vi "HB_Society.Main.vi"() -> ()   [LabVIEW 2009, in "HB_BaseClass_Examples.lvlib"]
doc: "This is a VI to test the simple composition without usage of the Visitor Pattern.\n\nIt demonstrates how to build a continent with contries and towns."
uses:
  HB_BaseClass_Examples.lvlib
  HB_Factory/HB_Factory.lvclass
  HB_Society.lvclass
  lib.lib/HGF_LVC/HGF_BaseClasses/HGF_Factory/HGF_Factory.lvclass
  lib.lib/HGF_LVC/HGF_BaseClasses/HGF_Composite/HGF_Composite.lvclass
panel:
  out "objects":T1(array[cluster])
  out "nofPersons 3":dbl
  out "nofPersons 2":dbl
  out "nofPersons 1":dbl
  in  "Continent":string="Europe"
  in  "Countries":T2(array[cluster])=[{"Name"="Germany", "Towns"=[{"Name"="Essen", "nofPersons"=300}, {"Name"="Bochum", "nofPersons"=200}, {"Name"="Darmstadt", "nofPersons"=200}]}, {"Name"="Montenegro", "Towns"=[{"Name"="Podgorica", "nofPersons"=300}, {"Name"="Bar", "nofPersons"=200}, {"Name"="Ulcinj", "nofPersons"=100}]}]
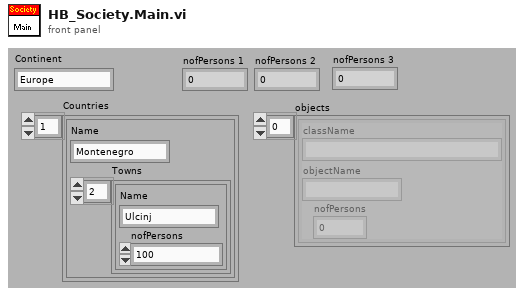
[diagram p1: front panel]
types:
  T1 = cluster{"className":string, "objectName":string, "nofPersons":dbl}[]
  T2 = cluster{"Name":string, "Towns":cluster{"Name":string, "nofPersons":i32}[]}[]
  T3 = cluster{"className":string, "objectName":string, "nofPersons":dbl}
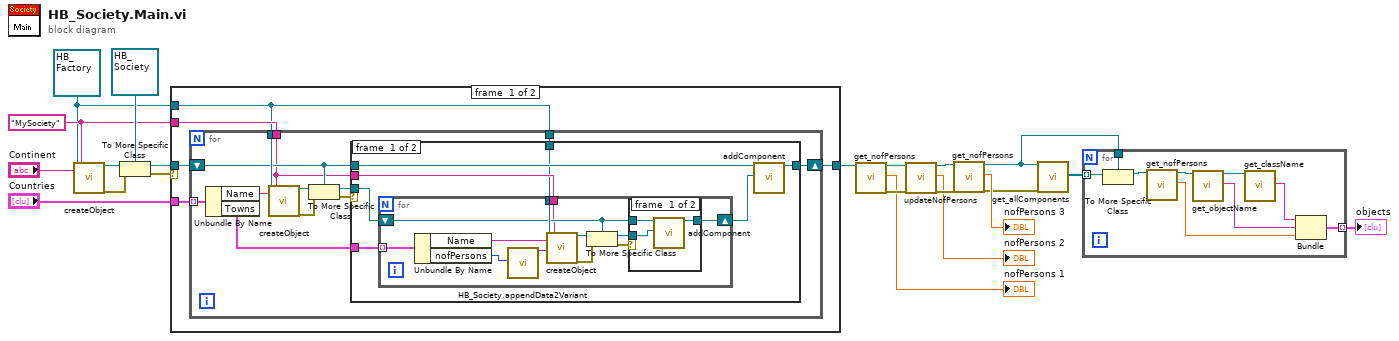
[diagram p0: block diagram]
diagram:
  w5 = "MySociety" ("className")
  w2 = refnum<class "HB_Factory.lvclass"> refnum ("HB_Factory.lvclass")
  n1 = call "createObject.vi"("HGF_Factory"=w2, "objectName"="Continent", "className"=w5) -> ("HGF_Object"=w1:refnum<class "HGF_Factory.lvclass">, "error out"=w3:errorcluster)  [unwired: 4 in, 11 out]
  n2 = To More Specific Class(target class=refnum<class "HB_Society.lvclass"> refnum ("MySociety.lvclass"), reference=w1, error in=w3) -> (specific class reference=w19:refnum<class "HB_Society.lvclass">, error out=w18:errorcluster)
  n3 = case shown="No Error" w18 {
    tunnel: "Countries" -> [w26 _]
    tunnel: w2 -> [w22 _]
    tunnel: w5 -> [w25 _]
    tunnel: w19 -> [w24 w63]
    tunnel: [w23 w63] -> w14
    frame #0 {
      n4 = for {
        tunnel: w22 -> [w36]
        tunnel: w26 -> [w38] mode=indexing
        tunnel: w25 -> [w31]
        shift-right: [w32] -> w23
        shift-left: w24 -> [w33]
        tunnel: w22 -> [w29]
        n5 = Unbundle By Name(w38) -> ("Name"=w30:string, "Towns"=w37:cluster{"Name":string, "nofPersons":i32}[])
        n6 = call "createObject.vi"("HGF_Factory"=w36, "objectName"=w30, "className"=w31) -> ("HGF_Object"=w28:refnum<class "HGF_Factory.lvclass">, "error out"=w27:errorcluster)  [unwired: 3 in, 12 out]
        n7 = To More Specific Class(target class=w33, reference=w28, error in=w27) -> (specific class reference=w35:refnum<class "HB_Society.lvclass">, error out=w34:errorcluster)
        n8 = case shown="No Error" w34 {
          tunnel: w37 -> [w45 _]
          tunnel: w31 -> [w44 _]
          tunnel: w35 -> [w43 _]
          tunnel: w33 -> [w42 w62]
          tunnel: [w40 w62] -> w32
          tunnel: w29 -> [w39 _]
          frame #0 {
            n9 = for {
              tunnel: w39 -> [w57]
              tunnel: w45 -> [w56] mode=indexing
              tunnel: w44 -> [w51]
              shift-right: [w54] -> w41
              shift-left: w43 -> [w55]
              n10 = Unbundle By Name(w56) -> ("Name"=w50:string, "nofPersons"=w46:i32)
              n11 = call "HB_Society.appendData2Variant.vi"("nofPersons"=w46) -> ("dup initData"=w47:variant)  [unwired: 2 in, 16 out]
              n12 = call "createObject.vi"("HGF_Factory"=w57, "objectName"=w50, "initializationData"=w47, "className"=w51) -> ("HGF_Object"=w49:refnum<class "HGF_Factory.lvclass">, "error out"=w48:errorcluster)  [unwired: 2 in, 12 out]
              n13 = To More Specific Class(target class=w55, reference=w49, error in=w48) -> (specific class reference=w53:refnum<class "HB_Society.lvclass">, error out=w52:errorcluster)
              n14 = case shown="No Error" w52 {
                tunnel: w55 -> [w60 w61]
                tunnel: [w59 w61] -> w54
                tunnel: w53 -> [w58 _]
                frame #0 {
                  n15 = call "addComponent.vi"("HGF_Composite"=w60, "HGF_Component"=w58) -> ("dup HGF_Composite"=w59:refnum<class "HB_Society.lvclass">)  [unwired: 1 in, 16 out]
                }
                frame #1 {
                }
              }
            }
            n16 = call "addComponent.vi"("HGF_Composite"=w42, "HGF_Component"=w41) -> ("dup HGF_Composite"=w40:refnum<class "HB_Society.lvclass">)  [unwired: 1 in, 16 out]
          }
          frame #1 {
          }
        }
      }
    }
    frame #1 {
    }
  }
  n17 = call "get_nofPersons.vi"("MySociety"=w14) -> ("dup MySociety"=w15:refnum<class "HB_Society.lvclass">, "nofPersons"=→"nofPersons 1":dbl, "error out"=w16:errorcluster)  [unwired: 1 in, 15 out]
  n18 = call-dynamic "updateNofPersons.vi"("MySociety"=w15, "error in (no error)"=w16) -> ("dup MySociety"=w17:refnum<class "HB_Society.lvclass">, "nofPersons"=→"nofPersons 2":dbl, "error out"=w13:errorcluster)  [unwired: 15 out]
  n19 = call "get_nofPersons.vi"("MySociety"=w17, "error in (no error)"=w13) -> ("dup MySociety"=w7:refnum<class "HB_Society.lvclass">, "nofPersons"=→"nofPersons 3":dbl, "error out"=w9:errorcluster)  [unwired: 15 out]
  n20 = call-dynamic "get_allComponents.vi"("HGF_Component in"=w7, "error in (no error)"=w9) -> ("Components"=w8:refnum<class "HGF_Component.lvclass">[])  [unwired: 17 out]
  n21 = for {
    tunnel: w8 -> [w72] mode=indexing
    tunnel: w7 -> [w70]
    tunnel: [w66] -> w6 mode=indexing
    n22 = To More Specific Class(target class=w70, reference=w72) -> (specific class reference=w71:refnum<class "HB_Society.lvclass">)  [unwired: 1 in, 1 out]
    n23 = call "get_nofPersons.vi"("MySociety"=w71) -> ("dup MySociety"=w69:refnum<class "HB_Society.lvclass">, "nofPersons"=w67:dbl)  [unwired: 1 in, 16 out]
    n24 = call "get_objectName.vi"("HGF_Factory"=w69) -> ("dup HGF_Factory"=w65:refnum<class "HB_Society.lvclass">, "objectName"=w68:string)  [unwired: 1 in, 16 out]
    n25 = call "get_className.vi"("HGF_Factory"=w65) -> ("className"=w64:string)  [unwired: 1 in, 17 out]
    n26 = Bundle("className"=w64, "objectName"=w68, "nofPersons"=w67) -> (w66:T3)  [unwired: 1 out]
  }
  "objects" <- w6
